vi "Revision Query.vi"(8 "error in (no error)":errorcluster, 11 "VISA resource name":refnum<visa-resource-name>) -> (0 "error out":errorcluster, 1 "Instr Firmware Revision":string, 2 "Instr Driver Revision":string, 3 "VISA resource name out":refnum<visa-resource-name>)   [LabVIEW 2017, in "Agilent 4194.lvlib"]
doc: "This VI queries the current instrument firmware revision and instrument driver revision. This Instrument Driver's Revision number is \"REV 1.0, 03/1999, LV 5.0.1\" and is compatible with Instrument Firmware Revision \"1.0\"\n\nNotes: \n(1) This instrument does not support an Firmware Revision and this VI will return a Warning if it is executed.\n\nHewlett-Packard 4194A Impedance/Gain-Phase Analyzer\nRelease Date: March 1999\nOriginally Developed in LabVIEW Version:5.0.1\nCreated By: Tom Wittassek\nTechnical University Ostrava\nDepartment of Electrical Measurement\nFaculty of Electrical Engineering and Informatics\nCzech Republic\nE-mail address: tomas.wittassek@vsb.cz\nModification History: \n\nNone"
uses:
  Agilent 4194.lvlib
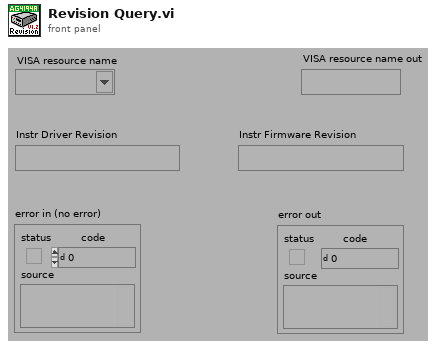
[diagram p1: front panel]
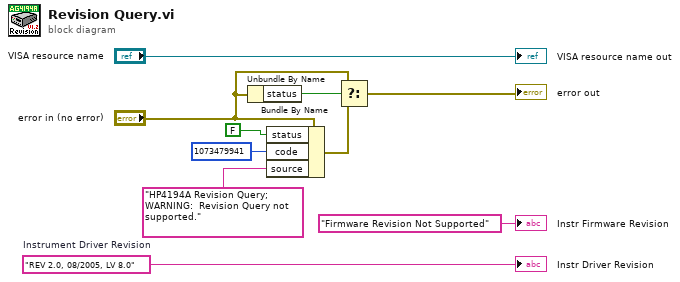
[diagram p0: block diagram]
diagram:
  w10 = "REV 2.0, 08/2005, LV 8.0"  # Instrument Driver Revision
  n1 = Unbundle By Name("error in (no error)") -> ("status"=w5:bool)
  n2 = Bundle By Name(cluster="error in (no error)", "status"=FALSE ("Status"), "code"=1073479941 ("Code"), "source"="HP4194A Revision Query; WARNING:  Revision Query not supported." ("Warning Message:")) -> (w4:errorcluster)
  n3 = Select(t="error in (no error)", s=w5, f=w4) -> (s? t:f=→"error out":errorcluster)
  "Instr Firmware Revision" <- "Firmware Revision Not Supported"
  "Instr Driver Revision" <- w10
  "VISA resource name out" <- "VISA resource name"
